vi "tm_getarea_a.vi"(8 "error in (no error)":errorcluster, 11 "Handle in":u32) -> (0 "error out":errorcluster, 1 "V Offset":T1, 2 "H Offset":T1, 3 "Handle out":u32, 4 "H Width":T1, 6 "V Width":T1)   [LabVIEW 2023]
uses:
  tmcamcon.dll
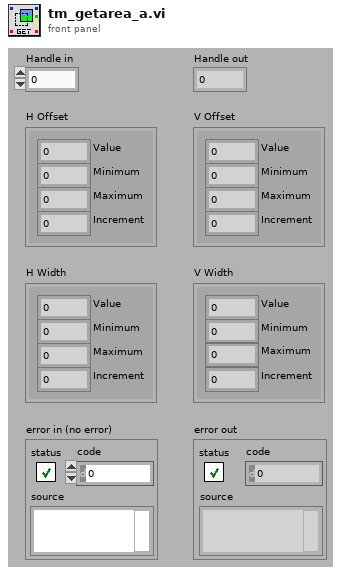
[diagram p1: front panel]
types:
  T1 = cluster{"Value":i32, "Minimum":i32, "Maximum":i32, "Increment":i32}
  T2 = cluster{"hov":i32, "hon":i32, "hox":i32, "hoi":i32}
  T3 = cluster{"hwv":i32, "hwn":i32, "hwx":i32, "hwi":i32}
  T4 = cluster{"vov":i32, "von":i32, "vox":i32, "voi":i32}
  T5 = cluster{"vwv":i32, "vwn":i32, "vwx":i32, "vwi":i32}
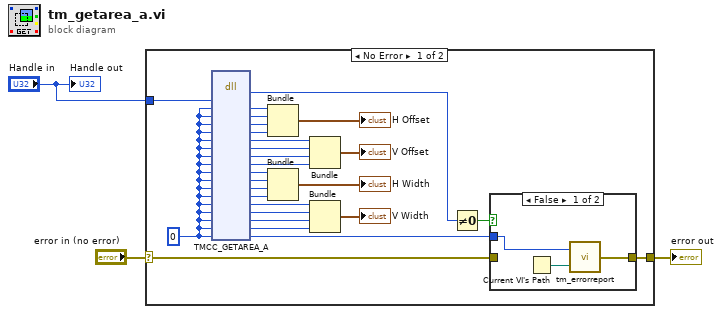
[diagram p0: block diagram]
diagram:
  n1 = case shown="No Error" "error in (no error)" {
    selector: "error in (no error)" -> [w7 w35]
    tunnel: [w4 w35] -> w2
    tunnel: "Handle in" -> [w8 _]
    frame No Error {
      w24 = 0
      n2 = dll-call lib="tmcamcon.dll" fn="TMCC_GETAREA_A"("index"=w8, "hov"=w24, "hon"=w24, "hox"=w24, "hoi"=w24, "vov"=w24, "von"=w24, "vox"=w24, "voi"=w24, "hwv"=w24, "hwn"=w24, "hwx"=w24, "hwi"=w24, "vwv"=w24, "vwn"=w24, "vwx"=w24, "vwi"=w24, "Erval"=w24) -> ("return type"=w30:u32, "hov"=w27:i32, "hon"=w28:i32, "hox"=w29:i32, "hoi"=w26:i32, "vov"=w23:i32, "von"=w22:i32, "vox"=w21:i32, "voi"=w20:i32, "hwv"=w19:i32, "hwn"=w18:i32, "hwx"=w17:i32, "hwi"=w16:i32, "vwv"=w15:i32, "vwn"=w14:i32, "vwx"=w13:i32, "vwi"=w12:i32, "Erval"=w5:i32)  [unwired: 4 in, 2 out]
      n3 = Bundle("hov"=w27, "hon"=w28, "hox"=w29, "hoi"=w26) -> (→"H Offset":T2)  [unwired: 1 in]
      n4 = Bundle("hwv"=w19, "hwn"=w18, "hwx"=w17, "hwi"=w16) -> (→"H Width":T3)  [unwired: 1 in]
      n5 = Bundle("vov"=w23, "von"=w22, "vox"=w21, "voi"=w20) -> (→"V Offset":T4)  [unwired: 1 in]
      n6 = Bundle("vwv"=w15, "vwn"=w14, "vwx"=w13, "vwi"=w12) -> (→"V Width":T5)  [unwired: 1 in]
      n7 = Not Equal To 0?(x=w30) -> (x != 0?=w6:bool)
      n8 = case shown="False" w6 {
        tunnel: w7 -> [_ w34]
        tunnel: [w32 w34] -> w4
        tunnel: w5 -> [w31 _]
        frame False {
          n9 = Current VI's Path() -> (path=w33:path)
          n10 = call "tm_errorreport.vi"("Source"=w33, "Error"=w31) -> ("error out"=w32:errorcluster)
        }
        frame True {
        }
      }
    }
    frame Error {
    }
  }
  "error out" <- w2
  "Handle out" <- "Handle in"
